vi "Unit test-AVI frame rate PID control.vi"() -> ()   [LabVIEW 2017]
uses:
  User Interface/Visualisation/Timelapse Viewer/Globals/gl_Time series viewer globals.vi
panel:
  in  "integral time (Ti, min)":dbl=0.01 min=0.0 max=2142532154361346.0 step=0.01 format="%#_13g"
  in  "proportional gain (Kc)":dbl=0.7 min=0.0 step=0.05 format="%#_13g"
  in  "Frame period (ms)":u32=75
  in  "Delay":u32
  out "Required frame rate (fps)":dbl
  out "Actual frame rate (fps)":dbl
  out "Chart":cluster{dbl, dbl}(graph) caption="Frame rate (fps)"
  out "Actual frame period (ms)":u32
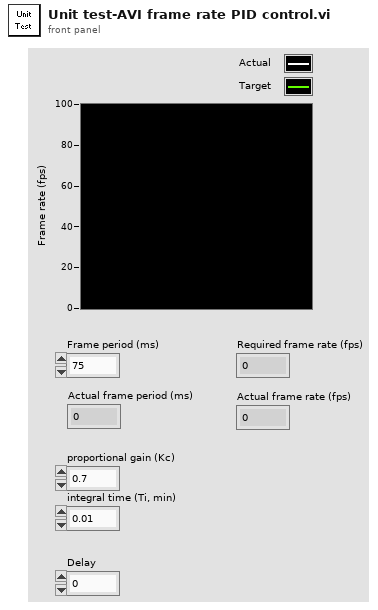
[diagram p1: front panel]
types:
  T1 = typedef "AVI playback header info cluster.ctl" = cluster{"Frame Size":u32, "AOD fill time (us)":dbl, "Dwell time (us)":dbl, "Frame period (ms)":dbl, "Number of Miniscans":u16, "Number of Pixels in Miniscan":u16}
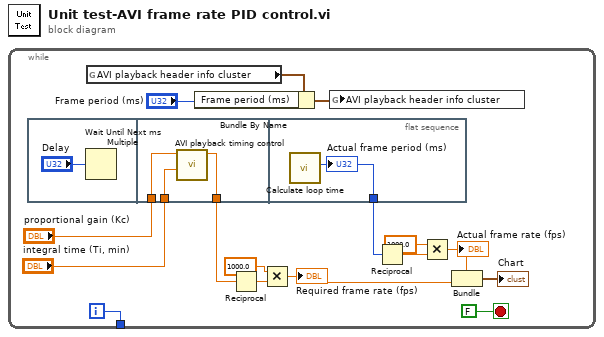
[diagram p0: block diagram]
diagram:
  n1 = while {
    tunnel: [w15] -> _
    i -> [w15]
    stop <- FALSE stop-if-true
    n2 = flat-sequence {
      tunnel: [w20] -> w14
      tunnel: "proportional gain (Kc)" -> [w19]
      tunnel: "integral time (Ti, min)" -> [w18]
      tunnel: [w21] -> w13
      frame #0 {
        n3 = Wait Until Next ms Multiple(millisecond multiple="Delay") -> ()  [unwired: 1 out]
      }
      frame #1 {
        n4 = call "AVI playback timing control.vi"("integral time (Ti, min)"=w18, "proportional gain (Kc)"=w19) -> ("Original frame rate (fps)"=w20:dbl)  [unwired: 6 in, 3 out]
      }
      frame #2 {
        n5 = call <userlib>:"Calculate loop time.vi"() -> ("Loop time (ms)"=w21:u32)  [unwired: 11 in]
        "Actual frame period (ms)" <- w21
      }
    }
    n6 = global read "gl_Time series viewer globals.vi" "AVI playback header info cluster"() -> (w5:T1)
    n7 = Bundle By Name(cluster=w5, "Frame period (ms)"="Frame period (ms)") -> (w4:T1)
    n8 = Reciprocal(x=w14) -> (1/x=w11:dbl)
    n9 = Multiply(x=1000.0, y=w11) -> (x*y=w7:dbl)
    "Required frame rate (fps)" <- w7
    n10 = global write "gl_Time series viewer globals.vi" "AVI playback header info cluster"(w4) -> ()
    n11 = Reciprocal(x=w13) -> (1/x=w12:dbl)
    n12 = Multiply(x=1000.0, y=w12) -> (x*y=w8:dbl)
    "Actual frame rate (fps)" <- w8
    n13 = Bundle(w8, w7) -> (→"Chart":cluster{dbl, dbl})  [unwired: 1 in]
  }
